vi "parse_return_serial.vi"(11 "string":string) -> (3 "Status":T1)   [LabVIEW 2019]
uses:
  status_cluster_typedef.ctl
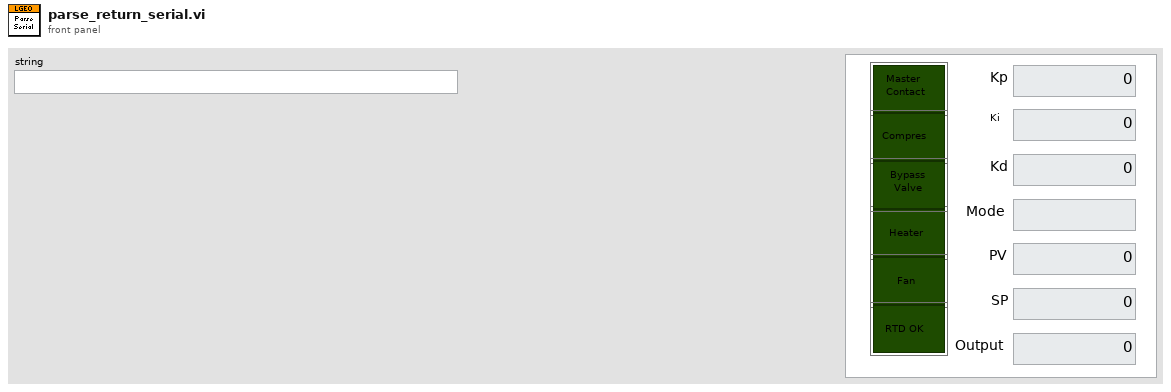
[diagram p1: front panel]
types:
  T1 = typedef "status_cluster_typedef.ctl" = cluster{"Master\nContact":bool, "Heater":bool, "Fan":bool, "Compres":bool, "Bypass\nValve":bool, "Kp":dbl, "Ki":dbl, "Kd":dbl, "Mode":string, "PV":dbl, "SP":dbl, "RTD OK":bool, "Output":dbl}
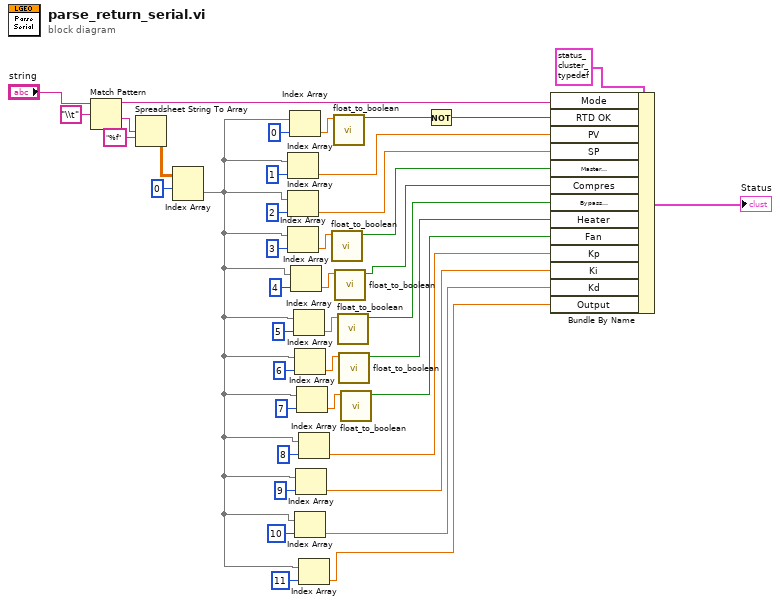
[diagram p0: block diagram]
diagram:
  n1 = Match Pattern(string="string", regular expression="\\t") -> (before substring=w38:string, after substring=w37:string)  [unwired: 1 in, 2 out]
  n2 = Spreadsheet String To Array(format string="%f", spreadsheet string=w37) -> (array=w36:dbl[][])  [unwired: 2 in]
  n3 = Index Array(array=w36, index (row)=0) -> (element=w8:dbl[])  [unwired: 1 in]
  n4 = Index Array(array=w8, index=1) -> (element=w31:dbl)
  n5 = Index Array(array=w8, index=2) -> (element=w29:dbl)
  n6 = Index Array(array=w8, index=3) -> (element=w13:dbl)
  n7 = Index Array(array=w8, index=0) -> (element=w34:dbl)
  n8 = Index Array(array=w8, index=4) -> (element=w14:dbl)
  n9 = Index Array(array=w8, index=5) -> (element=w15:dbl)
  n10 = Index Array(array=w8, index=6) -> (element=w16:dbl)
  n11 = Index Array(array=w8, index=10) -> (element=w5:dbl)
  n12 = Index Array(array=w8, index=9) -> (element=w6:dbl)
  n13 = Index Array(array=w8, index=7) -> (element=w17:dbl)
  n14 = Index Array(array=w8, index=8) -> (element=w7:dbl)
  n15 = Index Array(array=w8, index=11) -> (element=w4:dbl)
  n16 = call "float_to_boolean.vi"("Numeric"=w13) -> ("Boolean"=w27:bool)  [unwired: 10 in]
  n17 = call "float_to_boolean.vi"("Numeric"=w34) -> ("Boolean"=w1:bool)  [unwired: 10 in]
  n18 = call "float_to_boolean.vi"("Numeric"=w14) -> ("Boolean"=w26:bool)  [unwired: 10 in]
  n19 = call "float_to_boolean.vi"("Numeric"=w15) -> ("Boolean"=w25:bool)  [unwired: 10 in]
  n20 = call "float_to_boolean.vi"("Numeric"=w16) -> ("Boolean"=w24:bool)  [unwired: 10 in]
  n21 = call "float_to_boolean.vi"("Numeric"=w17) -> ("Boolean"=w23:bool)  [unwired: 10 in]
  n22 = Not(x=w1) -> (.not. x?=w2:bool)
  n23 = Bundle By Name(cluster=T1 {"Master\nContact"=FALSE, "Heater"=FALSE, "Fan"=FALSE, "Compres"=FALSE, "Bypass\nValve"=FALSE, "Kp"=0.0, "Ki"=0.0, "Kd"=0.0, "Mode"="", "PV"=0.0, "SP"=0.0, "RTD OK"=FALSE, "Output"=0.0} ("Status"), "Mode"=w38, "RTD OK"=w2, "PV"=w31, "SP"=w29, "Master\nContact"=w27, "Compres"=w26, "Bypass\nValve"=w25, "Heater"=w24, "Fan"=w23, "Kp"=w7, "Ki"=w6, "Kd"=w5, "Output"=w4) -> (→"Status":T1)
